vi "Util_HoodPositionCalculations.vi"(11 "Sonar Distance":dbl) -> (3 "Hood Position":dbl)   [LabVIEW 2017, in "Shooter.lvlib"]
uses:
  Shooter.lvlib
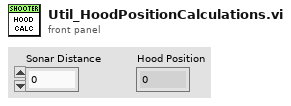
[diagram p1: front panel]
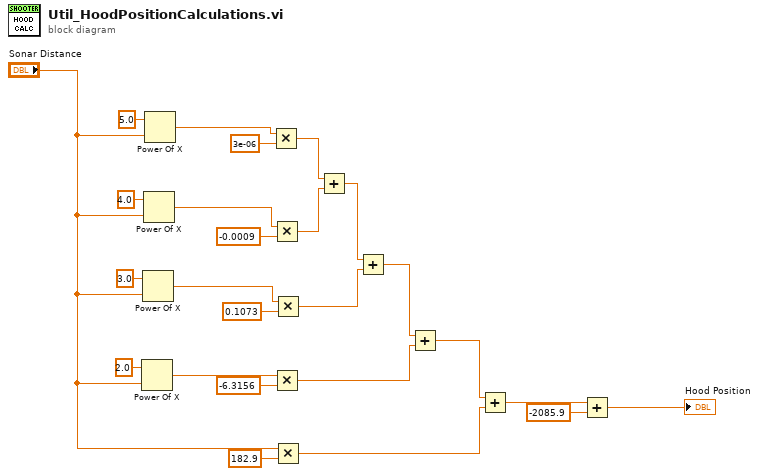
[diagram p0: block diagram]
diagram:
  n1 = Power Of X(1:"Sonar Distance", 2:2.0 ("y")) -> (0:w5:dbl)
  n2 = Power Of X(1:"Sonar Distance", 2:3.0 ("y")) -> (0:w20:dbl)
  n3 = Power Of X(1:"Sonar Distance", 2:4.0 ("y")) -> (0:w21:dbl)
  n4 = Power Of X(1:"Sonar Distance", 2:5.0 ("y")) -> (0:w22:dbl)
  n5 = Multiply(x=w22, y=3e-06) -> (x*y=w15:dbl)
  n6 = Multiply(x=w21, y=-0.0009) -> (x*y=w14:dbl)
  n7 = Multiply(x=w5, y=-6.3156) -> (x*y=w10:dbl)
  n8 = Multiply(x=w20, y=0.1073) -> (x*y=w12:dbl)
  n9 = Multiply(x="Sonar Distance", y=182.9) -> (x*y=w6:dbl)
  n10 = Add(x=w15, y=w14) -> (x+y=w13:dbl)
  n11 = Add(x=w13, y=w12) -> (x+y=w11:dbl)
  n12 = Add(x=w11, y=w10) -> (x+y=w8:dbl)
  n13 = Add(x=w8, y=w6) -> (x+y=w7:dbl)
  n14 = Add(x=w7, y=-2085.9) -> (x+y=→"Hood Position":dbl)
